vi "Read Subscribed Topics.vi"(8 "error in (no error)":errorcluster) -> (0 "error out":errorcluster)   [LabVIEW 2020, in "DAQIO MQTT.lvlib"]
doc: "A basic example that reads topics that the client subcribed to. \n\n© 2015 - daq.io, LLC - Peter Adelhardt"
uses:
  DAQIO MQTT.lvlib
  Controls/Connect Flags.ctl
  Controls/Retain_Flag.ctl
  Controls/DUP Flag.ctl
  Controls/User Info.ctl
  Controls/Connection Return Codes.ctl
panel:
  out "Connection Status":T1=enum."Connection refused: not authorized"
  in  "Exit":bool
  in  "MQTT Broker":cluster{"address (IP)":string, "port":u16}={"address (IP)"="broker.hivemq.com", "port"=1883}
  out "Topics":string[](array[string])
  out "Messages":string[](array[string])
  in  "Client ID":string="LVSubscribeClient"
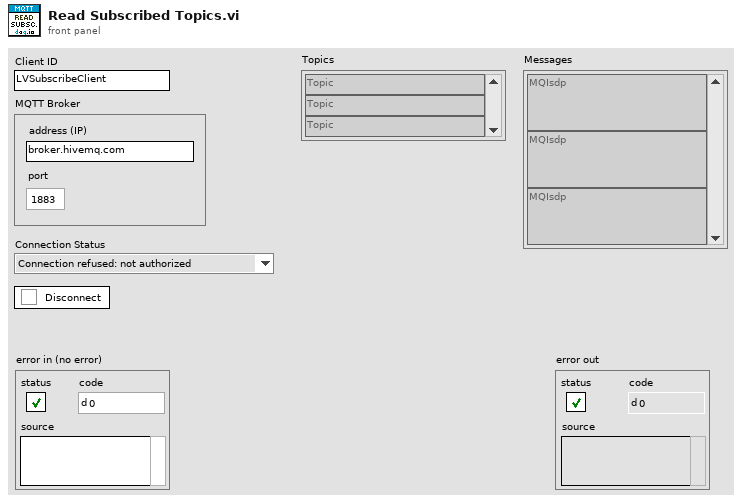
[diagram p1: front panel]
types:
  T1 = typedef "DAQIO MQTT.lvlib/Connection Return Codes.ctl" = enum16{"Connection accepted", "Connection refused: unacceptable protocol version", "Connection refused: identifier rejected", "Connection refused: Server unavailable", "Connection refused: bad user name or password", "Connection refused: not authorized"}
  T2 = typedef "DAQIO MQTT.lvlib/User Info.ctl" = cluster{"Username":string, "Password":string}
  T3 = typedef "DAQIO MQTT.lvlib/DUP Flag.ctl" = bool
  T4 = typedef "DAQIO MQTT.lvlib/Retain_Flag.ctl" = bool
  T5 = cluster{"QoS":enum8{"At most once", "At least once", "Exactly once", "Reserved"}, "DUP":T3, "Retain":T4, "Keep Alive (sec)":u16}
  T6 = typedef "DAQIO MQTT.lvlib/Connect Flags.ctl" = cluster{"user name":bool, "password":bool, "will retain":bool, "will flag":bool, "clean session":bool, "reserved":bool, "will QoS":enum8{"At most once", "At least once", "Exactly once", "Reserved"}}
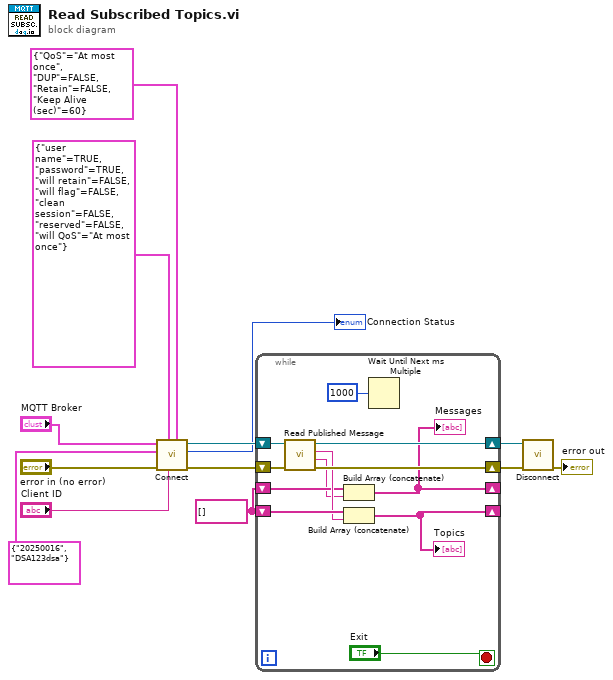
[diagram p0: block diagram]
diagram:
  w6 = string[] []
  n1 = call "Connect.vi"("Connect Meta"=T5 {"QoS"=enum."At most once", "DUP"=FALSE, "Retain"=FALSE, "Keep Alive (sec)"=60}, "Client ID"="Client ID", "Connect Flags"=T6 {"user name"=TRUE, "password"=TRUE, "will retain"=FALSE, "will flag"=FALSE, "clean session"=FALSE, "reserved"=FALSE, "will QoS"=enum."At most once"}, "error in (no error)"="error in (no error)", "User Info"=T2 {"Username"="20250016", "Password"="DSA123dsa"}, "MQTT Broker"="MQTT Broker") -> ("error out"=w2:errorcluster, "Connection Status"=→"Connection Status":T1, "connection ID out"=w4:refnum<k5>)  [unwired: 3 in]
  n2 = while {
    shift-right: [w20] -> w8
    shift-left: w2 -> [w22]
    shift-right: [w14] -> _
    shift-left: w6 -> [w17]
    shift-right: [w15] -> _
    shift-left: w6 -> [w19]
    shift-right: [w21] -> w9
    shift-left: w4 -> [w23]
    stop <- "Exit" stop-if-true
    n3 = call "Read Published Message.vi"("error in (no error)"=w22, "connection ID"=w23) -> ("error out"=w20:errorcluster, "Message"=w16:string, "Topic"=w18:string, "connection ID out"=w21:refnum<k5>)  [unwired: 6 in]
    n4 = Build Array (concatenate)(w17, w16) -> (w14:string[])
    "Messages" <- w14
    n5 = Build Array (concatenate)(w19, w18) -> (w15:string[])
    "Topics" <- w15
    n6 = Wait Until Next ms Multiple(millisecond multiple=u32 1000) -> ()  [unwired: 1 out]
  }
  n7 = call "Disconnect.vi"("error in (no error)"=w8, "connection ID"=w9) -> ("error out"=→"error out":errorcluster)  [unwired: 9 in]
